vi "Send Configure Multi-Point [MP].vi"(5 "sample interval (0.0 s)":dbl format="%.3f", 6 "sample trigger (Immediate)":i32(ring)=1 items=["Immediate"=1, "External"=2, "Software Trigger Function"=3, "Interval"=10, "PXI TRIG0 or VXI TTL0"=111, "PXI TRIG1 or VXI TTL1"=112, "PXI TRIG2 or VXI TTL2"=113, "PXI TRIG3 or VXI TTL3"=114, "PXI TRIG4 or VXI TTL4"=115, "PXI TRIG5 or VXI TTL5"=116, "PXI TRIG6 or VXI TTL6"=117, "PXI TRIG7 or VXI TTL7"=118, "ECL0"=119, "ECL1"=120, "PXI Star"=131, "RTSI 0"=140, "RTSI 1"=141, "RTSI 2"=142, "RTSI 3"=143, "RTSI 4"=144, "RTSI 5"=145, "RTSI 6"=146], 7 "Message Priority (Normal)":T1=enum."Normal", 8 "error in (no error)":errorcluster, 9 "sample count (1)":i32=1, 10 "trigger count (1)":i32=1, 11 "Message Enqueuer":refnum<class "Message Enqueuer.lvclass">) -> (0 "error out":errorcluster, 3 "Message Enqueuer out":refnum<class "Message Enqueuer.lvclass">)   [LabVIEW 2015, in "CS++DMM.lvlib" / "Configure Multi-Point [MP] Msg.lvclass"]
doc: "Sends the <B>CS++DMM.lvlib:Configure Multi-Point [MP] Msg.lvclass</B> message.\n\n<B>CS++DMM.lvlib:CS++DMM.lvclass:Configure Multi-Point [MP].vi</B> Description:\n\nThis VI configures the properties that affect multi-point measurements. These properties are the trigger count, sample count, sample trigger and sample interval.\n\nNote:\n\n(1) This VI is part of the IviDmmMultiPoint [MP] extension group."
uses:
  Configure Multi-Point [MP] Msg.lvclass
  <vilib>/ActorFramework/Message Enqueuer/Message Enqueuer.lvclass
  <vilib>/ActorFramework/Message Enqueuer/Message Priority.ctl
  Configure Multi-Point [MP] Msg.lvclass/Configure Multi-Point [MP] Msg.ctl
  <vilib>/ActorFramework/Message Enqueuer/Message Enqueuer.lvclass/Message Enqueuer.ctl
  <vilib>/ActorFramework/Message Priority Queue/Priority Enqueue.vi
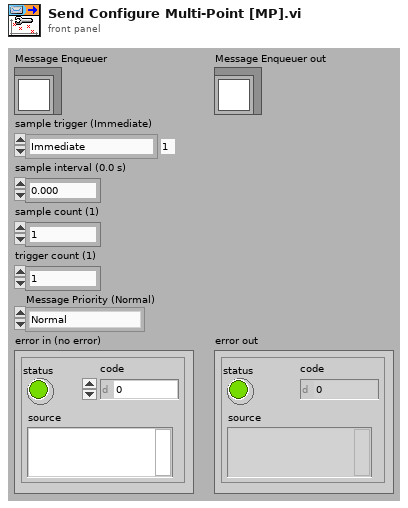
[diagram p1: front panel]
types:
  T1 = typedef "Actor Framework.lvlib/Message Enqueuer.lvclass/Message Priority.ctl" = enum16{"Low", "Normal", "High"}
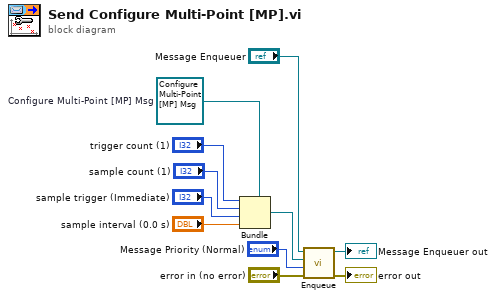
[diagram p0: block diagram]
diagram:
  w5 = refnum<class "Configure Multi-Point [MP] Msg.lvclass"> refnum  # Configure Multi-Point [MP] Msg
  n1 = Bundle(cluster=w5, "trigger count (1)", "sample count (1)", "sample trigger (Immediate)", "sample interval (0.0 s)") -> (w8:refnum<class "Configure Multi-Point [MP] Msg.lvclass">)
  n2 = call <vilib>:"Enqueue.vi"("error in (no error)"="error in (no error)", "Message Priority (Normal)"="Message Priority (Normal)", "Message"=w8, "Message Enqueuer in"="Message Enqueuer") -> ("error out"=→"error out":errorcluster, "Message Enqueuer out"=→"Message Enqueuer out":refnum<class "Message Enqueuer.lvclass">)  [unwired: 6 in]
